vi "HostDataNamesGLOBAL (1).vi"() -> ()   [LabVIEW 2017]
panel:
  out "Labels":string[](array[string])
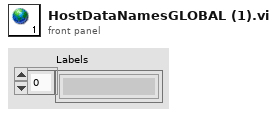
[diagram p1: front panel]
diagram:
